vi "Creator Queue Alias.vi"(11 "Template Queue in":refnum<class "Template Queue.lvclass">) -> (2 "Creator Queue Alias":string, 3 "Template Queue out":refnum<class "Template Queue.lvclass">)   [LabVIEW 2021, in "_Template.lvlib" / "Templates.lvlib" / "Template Queue.lvlib" / "Template Queue.lvclass"]
uses:
  Template Queue.lvclass
  Template Queue.lvclass/Template Queue.ctl
  <vilib>/jettl/jettl/jettl/Queue/Queue.lvclass
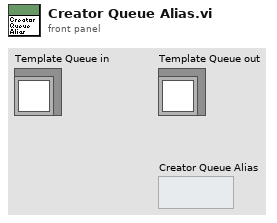
[diagram p1: front panel]
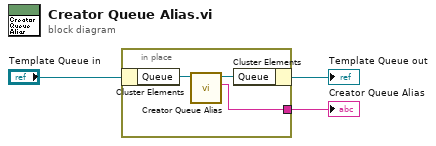
[diagram p0: block diagram]
diagram:
  n1 = in-place {
    in-place-border: [w5] -> w1
    n2 = in-place-cluster #1("Template Queue in") -> ("Queue"=w6:refnum<class "Queue.lvclass">)
    n3 = call-dynamic "Creator Queue Alias.vi"("Queue in"=w6) -> ("Creator Queue Alias"=w5:string, "Queue out"=w4:refnum<class "Queue.lvclass">)  [unwired: 9 in]
    n4 = in-place-cluster #1("Queue"=w4) -> (→"Template Queue out":refnum<class "Template Queue.lvclass">)
  }
  "Creator Queue Alias" <- w1
